vi "set in plane position.vi"(10 "Value":dbl, 11 "Instrument":T1 {"Input (1;B)" items=["A", "B"]; "Input (0:A) 325" items=["A", "B"]; "Input (0:A)" items=["A", "B"]; "Heater Output (1:1)" items=["1"=1, "2"=2]}) -> ()   [LabVIEW 2019, in "9T cmag.lvlib"]
uses:
  9T cmag.lvlib
  ctl/Instrument.ctl
  <vilib>/NI/Modbus Library/API/Master/Modbus Master.lvclass
  ctl/Instrument Type.ctl
  lib/QDInstrument.dll
  ctl/335 state.ctl
  ctl/limit.ctl
  ctl/9T mag field stauts.ctl
  User lib.lvlib
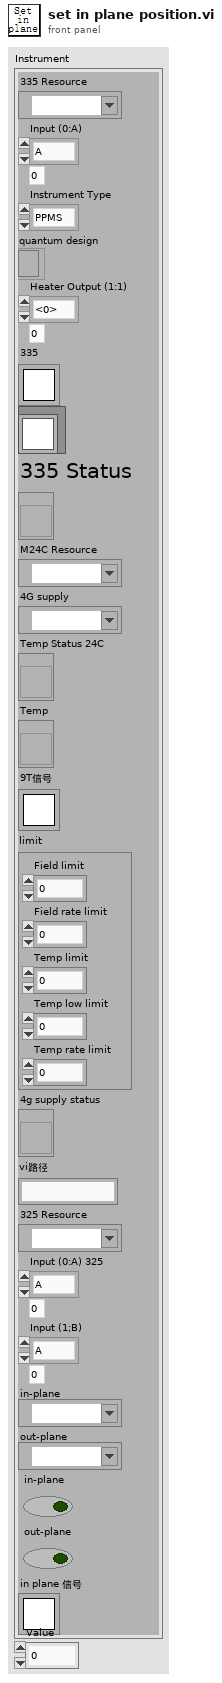
[diagram p1: front panel]
types:
  T1 = typedef "Instrument.ctl" = cluster{"335 Resource":refnum<visa-resource-name>, "Input (0:A)":u16, "Instrument Type":T2, "quantum design":refnum<k24>, "Heater Output (1:1)":u16, "semaphore":T3, "TCP master instance":refnum<class "Modbus Master.lvclass">, "335 Status":refnum<vi>, "M24C Resource":refnum<visa-resource-name>, "4G supply":refnum<visa-resource-name>, "Temp Status 24C":refnum<vi>, "Temp":refnum<vi>, "9T信号":T3, "limit":T4, "4g supply status":refnum<vi>, "vi路径":string, "325 Resource ":refnum<visa-resource-name>, "Input (0:A) 325":u16, "Input (1;B)":u16, "in-plane":refnum<visa-resource-name>, "out-plane":refnum<visa-resource-name>, "in-plane":bool, "out-plane":bool, "in plane 信号":T3}
  T2 = typedef "Instrument Type.ctl" = enum16{"PPMS", "VersaLab", "DynaCool", "SVSM", "PPMS-Rotate", "Lakeshore335", "9T mag"}
  T3 = typedef "Semaphore RefNum" = refnum<k1>
  T4 = typedef "limit.ctl" = cluster{"Field limit":dbl, "Field rate limit":dbl, "Temp limit":dbl, "Temp low limit":dbl, "Temp rate limit ":dbl}
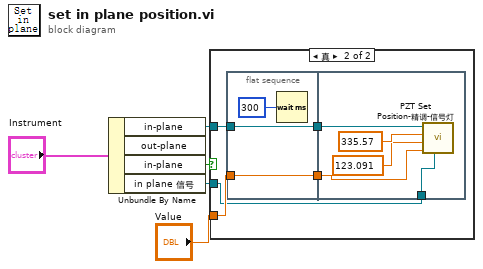
[diagram p0: block diagram]
diagram:
  n1 = Unbundle By Name("Instrument") -> ("in-plane"=w5:refnum<visa-resource-name>, "in-plane"=w4:bool, "in plane 信号"=w1:T3)  [unwired: 1 out]
  n2 = case shown="真" w4 {
    tunnel: "Value" -> [_ w10]
    tunnel: w5 -> [_ w9]
    tunnel: w1 -> [_ w8]
    frame False {
    }
    frame True {
      n3 = flat-sequence {
        tunnel: w9 -> [w12]
        tunnel: w10 -> [w13]
        tunnel: [w13] -> w7
        tunnel: [w12] -> w6
        tunnel: w8 -> [w14]
        tunnel: w7 -> [w16]
        tunnel: w6 -> [w15]
        frame #0 {
          n4 = Wait (ms)(milliseconds to wait=u32 300) -> ()  [unwired: 1 out]
        }
        frame #1 {
          n5 = call "PZT Set Position-精调-信号灯.vi"("in plane"=w14, "Set Position （°/mm）"=w16, "Origin"=123.091, "Range"=335.57, "VISA resource name"=w15) -> ()  [unwired: 4 in, 3 out]
        }
      }
    }
  }
